vi "Get TwinRX Coerced Configuration.vi"(0 "niUsrpRio Session":T3 {"Daughterboard Clock Rate" format="%#.3pHz"; "FPGA Data Clock Rate" format="%#.3pHz"; "Data Clock Rate" format="%#.3pHz"; "Characterization Data"."Frequencies [Hz]" format="%#_6p"; "EEPROM Characterization Header"."Pointer to Device Data Header" format="%x"; "EEPROM Characterization Header"."Checksum" format="%x"; "Device Data Header"."Pointer to Characterization Data" format="%x"; "Device Data Header"."Checksum" format="%x"; "EEPROM Header"."Pointer to User Header" format="%x"; "EEPROM Header"."Pointer to Factory Header" format="%x"; "EEPROM Header"."Product Code" format="%x"; "EEPROM Header"."Checksum" format="%x"}, 5 "rx.coerced configurations":T12, 11 "error in":errorcluster, 12 "rx config":T2={"channel configuration"=[], "transfer mode"=enum."Finite", "sample rate"=10000000.0, "number of samples"=8192, "start trigger"=enum."Immediate"} {"channel configuration"."channel configuration"."frequency" format="%#.3pHz"; "channel configuration"."channel configuration"."lo frequency" format="%#.3pHz"; "channel configuration"."channel configuration"."level" format="%#_gdBm"; "sample rate" format="%#.3pS/s"}) -> (4 "niUsrpRio Session (out)":T3 {"Daughterboard Clock Rate" format="%#.3pHz"; "FPGA Data Clock Rate" format="%#.3pHz"; "Data Clock Rate" format="%#.3pHz"; "Characterization Data"."Frequencies [Hz]" format="%#_6p"; "EEPROM Characterization Header"."Pointer to Device Data Header" format="%x"; "EEPROM Characterization Header"."Checksum" format="%x"; "Device Data Header"."Pointer to Characterization Data" format="%x"; "Device Data Header"."Checksum" format="%x"; "EEPROM Header"."Pointer to User Header" format="%x"; "EEPROM Header"."Pointer to Factory Header" format="%x"; "EEPROM Header"."Product Code" format="%x"; "EEPROM Header"."Checksum" format="%x"}, 6 "twinrx rx.coerced configurations":T13, 15 "error out":errorcluster)   [LabVIEW 2016]
uses:
  <instrlib>/niUsrpRio/Config/v1/Host/Public/niUsrpRio Session.ctl
  <instrlib>/_niInstr/Register Bus/v0/Host/Public/Register Bus Session.ctl
  <instrlib>/_niInstr/Register Bus/v0/Host/Private/Session Data.ctl
  <instrlib>/niUsrpRio/Config/v1/Host/Private/DB Queue Reference.ctl
  <instrlib>/niUsrpRio/Config/v1/Host/Private/Daughterboard Data.ctl
  <instrlib>/niUsrpRio/Config/v1/Host/Private/ATR state data.ctl
  <instrlib>/niUsrpRio/Config/v1/Host/Private/Antenna Configuration.ctl
  <instrlib>/niUsrpRio/Config/v1/Host/Private/CPLD Power Mode.ctl
  <instrlib>/niUsrpRio/Config/v1/Host/Public/EEPROM Header.ctl
  <instrlib>/niUsrpRio/Config/v1/Host/Public/EEPROM Device Data Header.ctl
  <instrlib>/niUsrpRio/Config/v1/Host/Public/EEPROM Characterization Header.ctl
  <instrlib>/niUsrpRio/Config/v1/Host/Public/Characterization Data.ctl
  <instrlib>/niUsrpRio/Config/v1/Host/Public/IQ Imbalance.ctl
  Start Trigger.ctl
  <instrlib>/niUsrpRio/Config/v1/Host/Private/TwinRX LO.ctl
  <instrlib>/niUsrpRio/Config/v1/Host/Private/niusrpriolv.lvlib
  <instrlib>/niUsrpRio/Config/v1/Host/niUsrpRio Config v1 Host.lvlib
  <instrlib>/_niInstr/Register Bus/v0/Host/niInstr Register Bus v0 Host.lvlib
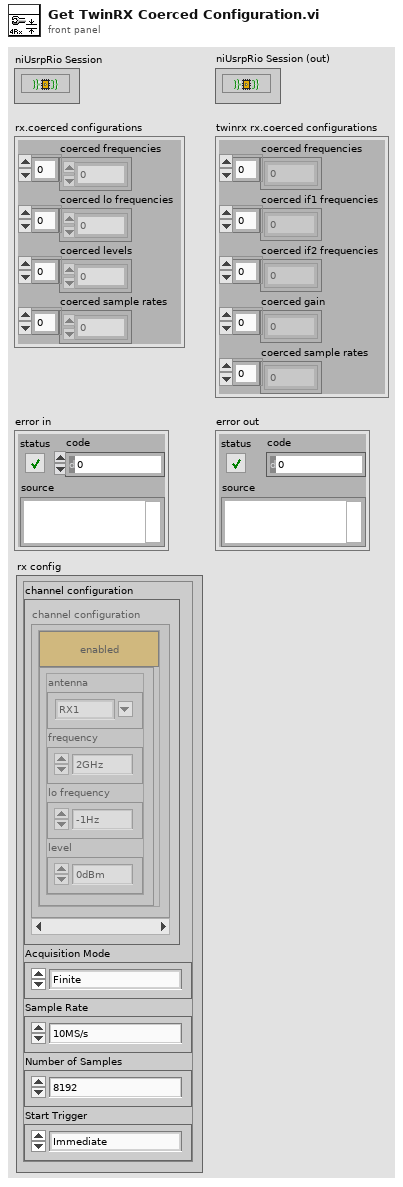
[diagram p1: front panel]
types:
  T1 = typedef "Start Trigger.ctl" = enum8{"Software", "Digital Edge", "Rx Start Trigger", "Tx Start Trigger", "Immediate", "Future Time Event"}
  T2 = cluster{"channel configuration":cluster{"channel enable":bool, "channel configuration":cluster{"antenna":string, "frequency":dbl, "lo frequency":dbl, "level":dbl}}[], "transfer mode":enum16{"Finite", "Continuous"}, "sample rate":dbl, "number of samples":u32, "start trigger":T1}
  T3 = typedef "niUsrpRio Config v1 Host.lvlib/niUsrpRio Session.ctl" = cluster{"FPGA Interface":refnum<k20>, "RIO Interface Number":u32, "Data Clock Rate":u32, "FPGA Data Clock Rate":u32, "Global Settings Register Bus":T4, "Radio 0 Settings Register Bus":T4, "Radio 1 Settings Register Bus":T4, "Radio Settings Bus Semaphore":T5, "DB Queues":T6[], "Characterization Data Valid?":bool, "EEPROM Header":T7, "Device Data Header":T8, "EEPROM Characterization Header":T9, "Characterization Data":T10[], "FPGA Current Version":u32, "FPGA Oldest Compatible Version":u32, "Fixed Logic Current Version":u32, "Fixed Logic Oldest Compatible Version":u32, "FPGA Radio Settings Bus Current Version":u32, "FPGA Radio Settings Bus Oldest Compatible Version":u32, "FPGA Board Config Current Version":u32, "FPGA Board Config Oldest Compatible Version":u32, "Daughterboard Clock Rate":u32, "daughterboard configuration session handles":u64[]}
  T4 = typedef "niInstr Register Bus v0 Host.lvlib/Register Bus Session.ctl" = refnum<queue>
  T5 = typedef "Semaphore RefNum" = refnum<k1>
  T6 = typedef "niUsrpRio Config v1 Host.lvlib/DB Queue Reference.ctl" = refnum<queue>
  T7 = typedef "niUsrpRio Config v1 Host.lvlib/EEPROM Header.ctl" = cluster{"Checksum":u32, "Product Code":u16, "Hardware Current Version":u16, "Hardware Oldest Compatible Version":u16, "EEPROM Map Current Version":u16, "EEPROM Map Oldest Compatible Version":u16, "User Password":string, "Pointer to Factory Header":u32, "Pointer to User Header":u32, "Recommended Interval":u16, "Number of Reserved Bytes":i32, "Number of Daughterboards":u8, "Daughterboard IDs":u16[], "Daughterboard Serial Numbers":string[]}
  T8 = typedef "niUsrpRio Config v1 Host.lvlib/EEPROM Device Data Header.ctl" = cluster{"Checksum":u32, "Number of Channels":u8, "Number of Gain Settings":u16[], "Pointer to Characterization Data":u32[], "Number of Reserved Bytes":i32, "Number of Frequencies":u16[]}
  T9 = typedef "niUsrpRio Config v1 Host.lvlib/EEPROM Characterization Header.ctl" = cluster{"Checksum":u32, "Date":timestamp, "Temperature":sgl, "Misc. Info":string, "Pointer to Device Data Header":u32, "Number of Reserved Bytes":i32}
  T10 = typedef "niUsrpRio Config v1 Host.lvlib/Characterization Data.ctl" = cluster{"Gains[dB]":dbl[], "Frequencies [Hz]":dbl[], "IQ Imbalance Table":T11[], "Measured Gains[dB]":dbl[][]}
  T11 = typedef "niUsrpRio Config v1 Host.lvlib/IQ Imbalance.ctl" = cluster{"Gain Imbalance [linear]":dbl, "Phase Imbalance [radians]":dbl, "Offset":cdb}
  T12 = cluster{"coerced frequencies":dbl[], "coerced lo frequencies":dbl[], "coerced levels":dbl[], "coerced sample rates":dbl[]}
  T13 = cluster{"coerced frequencies":dbl[], "coerced if1 frequencies":dbl[], "coerced if2 frequencies":dbl[], "coerced gain":dbl[], "coerced sample rates":dbl[]}
  T14 = cluster{"channel enable":bool, "channel configuration":cluster{"antenna":string, "frequency":dbl, "lo frequency":dbl, "level":dbl}}[]
  T15 = typedef "niUsrpRio Config v1 Host.lvlib/TwinRX LO.ctl" = enum16{"IF1", "IF2"}
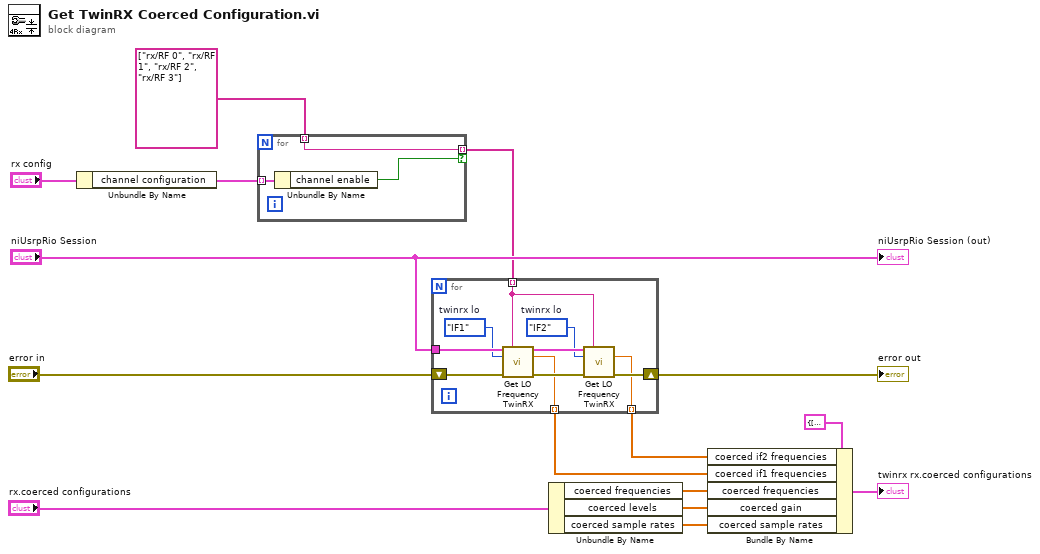
[diagram p0: block diagram]
diagram:
  n1 = Unbundle By Name("rx config") -> ("channel configuration"=w5:T14)
  n2 = for {
    tunnel: w5 -> [w18] mode=indexing
    tunnel: string[] ["rx/RF 0", "rx/RF 1", "rx/RF 2", "rx/RF 3"] -> [w17] mode=indexing
    tunnel: [w17] -> w3 mode=indexing if=w16
    n3 = Unbundle By Name(w18) -> ("channel enable"=w16:bool)
  }
  n4 = for {
    tunnel: "niUsrpRio Session" -> [w27]
    shift-right: [w23] -> w8
    shift-left: "error in" -> [w28]
    tunnel: w3 -> [w24] mode=indexing
    tunnel: [w22] -> w1 mode=indexing
    tunnel: [w19] -> w2 mode=indexing
    w20 = TwinRX_LO."IF2"  # twinrx lo
    w21 = TwinRX_LO."IF1"  # twinrx lo
    n5 = call <instrlib>:"Get LO Frequency TwinRX.vi"("niUsrpRio Session"=w27, "scope"=w24, "lo index"=w21, "error in"=w28) -> ("niUsrpRio Session (out)"=w26:T3, "frequency"=w19:dbl, "error out"=w25:errorcluster)  [unwired: 9 in]
    n6 = call <instrlib>:"Get LO Frequency TwinRX.vi"("niUsrpRio Session"=w26, "scope"=w24, "lo index"=w20, "error in"=w25) -> ("frequency"=w22:dbl, "error out"=w23:errorcluster)  [unwired: 9 in, 1 out]
  }
  "error out" <- w8
  n7 = Unbundle By Name("rx.coerced configurations") -> ("coerced frequencies"=w13:dbl[], "coerced levels"=w12:dbl[], "coerced sample rates"=w11:dbl[])
  n8 = Bundle By Name(cluster=T13 {"coerced frequencies"=[], "coerced if1 frequencies"=[], "coerced if2 frequencies"=[], "coerced gain"=[], "coerced sample rates"=[]} ("rx.coerced configurations"), "coerced if2 frequencies"=w1, "coerced if1 frequencies"=w2, "coerced frequencies"=w13, "coerced gain"=w12, "coerced sample rates"=w11) -> (→"twinrx rx.coerced configurations":T13)
  "niUsrpRio Session (out)" <- "niUsrpRio Session"
